vi "OpenLVProject.vi"(0 "Application ref":refnum<vi>, 1 "Project Path":path, 3 "error in":errorcluster) -> (7 "Application ref out":refnum<vi>, 8 "Project ref out":refnum<vi>, 10 "error out":errorcluster)   [LabVIEW 2017]
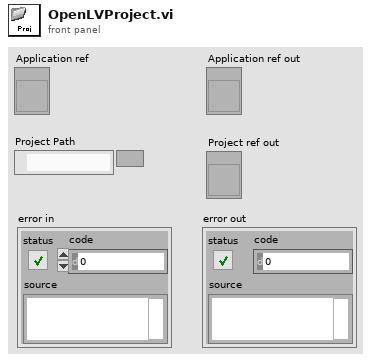
[diagram p1: front panel]
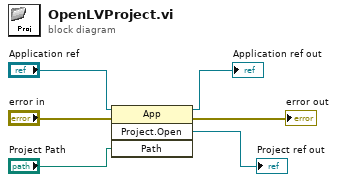
[diagram p0: block diagram]
diagram:
  n1 = invoke class="App" method="Project.Open"(reference="Application ref", error in="error in", "Path"="Project Path") -> (reference out=→"Application ref out":refnum<vi>, error out=→"error out":errorcluster, "Project:Open"=→"Project ref out":refnum<vi>)  [unwired: 1 in, 1 out]
